vi "LT_get_status.vi"(8 "error in":errorcluster, 10 "dev_param_in":T3={"Length of data block (14)"=14, "Converter address (0)"=0, "Converter type\n(180: Turbovac 350/450 i)"=180, "PZD1 STW, ZSW (0)"=0, "PZD2 HSW, HIW (0)"=0} {"Converter type\n(180: Turbovac 350/450 i)" items=["Turbovac 350/450 i"=180, "Turbovac 350/450 i with optional interface"=181, "Turbovac 350/450 iX"=182, "Turbovac  90/250 i"=190, "Turbovac  90/250 with optional interface"=191, "Turbovac  90/250 iX"=192, "Turbovac  850/950 i"=195, "Turbovac  850/950 i with optional interface"=196, "Turbovac  850/950 iX"=197, "Turbovac 1350/1450 i"=185, "Turbovac 1350/1450 i with optional interface"=186, "Turbovac 1350/1450 iX"=187]; "Length of data block (14)" items=["14"=14, "22"=22]}, 11 "VISA in":refnum<visa-resource-name>="COM43") -> (0 "error out":errorcluster, 1 "op_enabled":bool, 2 "dev_param_out":T5={"Length of data block"=14, "Converter address"=0, "Converter type"=180, "PZD1"=0, "PZD2"=0} {"Converter type" items=["Turbovac 350/450 i"=180, "Turbovac 350/450 i with optional interface"=181, "Turbovac 350/450 iX"=182, "Turbovac  90/250 i"=190, "Turbovac  90/250 with optional interface"=191, "Turbovac  90/250 iX"=192, "Turbovac  850/950 i"=195, "Turbovac  850/950 i with optional interface"=196, "Turbovac  850/950 iX"=197, "Turbovac 1350/1450 i"=185, "Turbovac 1350/1450 i with optional interface"=186, "Turbovac 1350/1450 iX"=187]; "Length of data block" items=["14"=14, "22"=22]}, 3 "VISA out":refnum<visa-resource-name>, 4 "status_error":u32(colorbox) caption="Status", 5 "Status values":T1, 6 "status_comm":bool caption="Comm. status", 7 "Status word":T2)   [LabVIEW 2019]
doc: "Example VI to demonstrate the use of the Oerlikon Leybold TMP driver."
uses:
  <instrlib>/Leybold TURBOVAC/Public/Ctl/Device Parameters Indicator.ctl
  <instrlib>/Leybold TURBOVAC/Public/Ctl/Converter Type Indicator.ctl
  <instrlib>/Leybold TURBOVAC/Public/Ctl/Device Parameters Control.ctl
  <instrlib>/Leybold TURBOVAC/Public/Ctl/Converter Type Control.ctl
  <instrlib>/Leybold TURBOVAC/Leybold TURBOVAC.lvlib
panel:
  out "Warnings / Errors":string
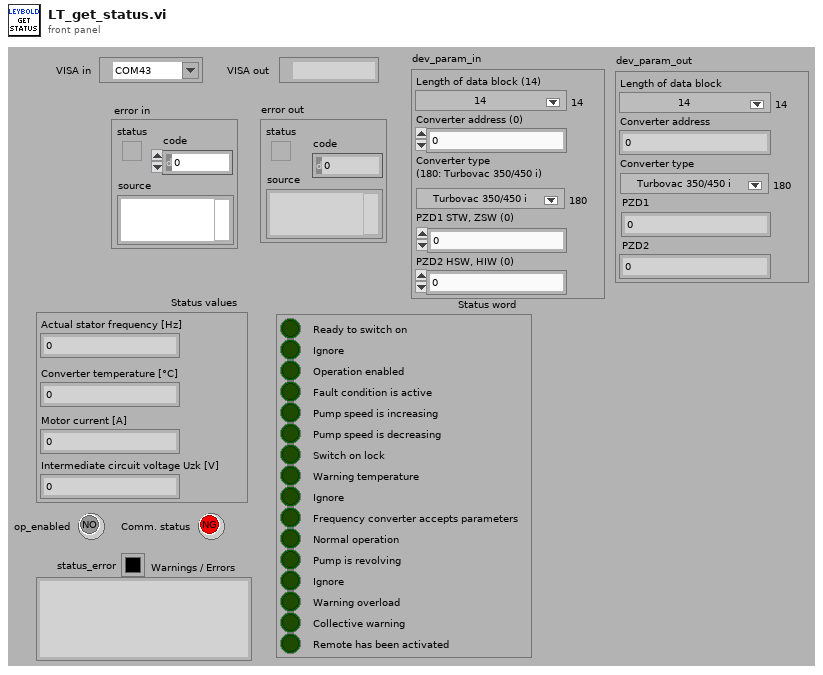
[diagram p1: front panel]
types:
  T1 = cluster{"Actual stator frequency [Hz]":u16, "Converter temperature [°C]":u16, "Motor current [A]":dbl, "Intermediate circuit voltage Uzk [V]":dbl}
  T2 = cluster{"Ready to switch on":bool, "Ignore":bool, "Operation enabled":bool, "Fault condition is active":bool, "Pump speed is increasing":bool, "Pump speed is decreasing":bool, "Switch on lock":bool, "Warning temperature":bool, "Ignore":bool, "Frequency converter accepts parameters":bool, "Normal operation":bool, "Pump is revolving":bool, "Ignore":bool, "Warning overload":bool, "Collective warning":bool, "Remote has been activated":bool}
  T3 = typedef "Leybold TURBOVAC.lvlib/Device Parameters Control.ctl" = cluster{"Length of data block (14)":u8, "Converter address (0)":u8, "Converter type\n(180: Turbovac 350/450 i)":T4, "PZD1 STW, ZSW (0)":u16, "PZD2 HSW, HIW (0)":u16}
  T4 = typedef "Leybold TURBOVAC.lvlib/Converter Type Control.ctl" = u16
  T5 = typedef "Leybold TURBOVAC.lvlib/Device Parameters Indicator.ctl" = cluster{"Length of data block":u8, "Converter address":u8, "Converter type":T6, "PZD1":u16, "PZD2":u16}
  T6 = typedef "Leybold TURBOVAC.lvlib/Converter Type Indicator.ctl" = u16
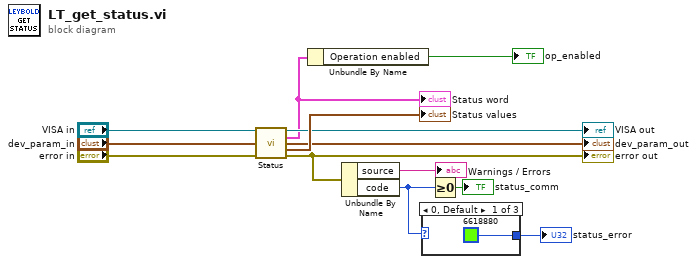
[diagram p0: block diagram]
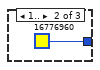
[diagram p2: hidden frame]
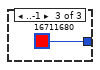
[diagram p3: hidden frame]
diagram:
  n1 = call <instrlib>:"Status.vi"("VISA resource name"="VISA in", "Device parameters"="dev_param_in", "error in (no error)"="error in") -> ("VISA resource name out"=→"VISA out":refnum<visa-resource-name>, "Status word"=w4:T2, "Device parameters out"=→"dev_param_out":T5, "Status values"=→"Status values":T1, "error out"=w6:errorcluster)  [unwired: 8 in]
  "error out" <- w6
  "Status word" <- w4
  n2 = Unbundle By Name(w4) -> ("Operation enabled"=→"op_enabled":bool)
  n3 = Unbundle By Name(w6) -> ("source"=→"Warnings / Errors":string, "code"=w2:i32)
  n4 = case shown="0, Default" w2 {
    tunnel: [u32 6618880 ("status_error") u32 16776960 ("status_error") u32 16711680 ("status_error")] -> w1
    frame 0, Default {
    }
    frame 1.. {
    }
    frame ..-1 {
    }
  }
  "status_error" <- w1
  n5 = Greater Or Equal To 0?(x=w2) -> (x >= 0?=→"status_comm":bool)
